vi "Read Auto update indicator.vi"(8 "error in (no error)":errorcluster, 11 "D_Datagrid in":refnum<class "D_Datagrid.lvclass">) -> (0 "error out":errorcluster, 2 "Auto-update indicator":bool, 3 "D_Datagrid out":refnum<class "D_Datagrid.lvclass">)   [LabVIEW 2018, in "D Datagrid Library.lvlib" / "D_Datagrid.lvclass"]
uses:
  D_Datagrid.lvclass
  D_Datagrid.lvclass/D_Datagrid.ctl
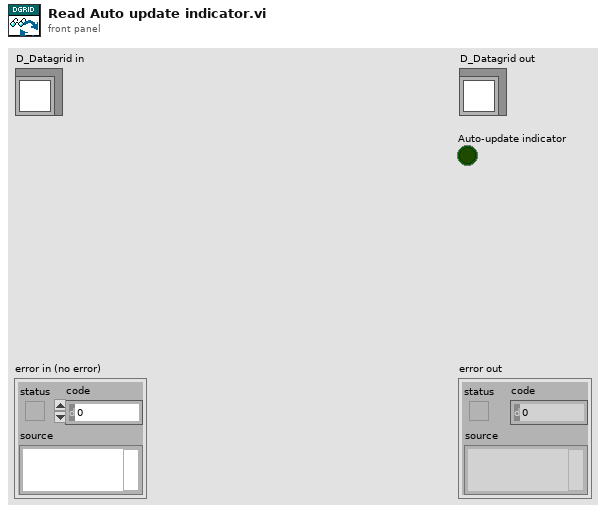
[diagram p1: front panel]
types:
  T1 = typedef "D Datagrid Library.lvlib/D_Datagrid.lvclass/State Data.ctl" = cluster{"Data elements":refnum<class "DatagridElement.lvclass">[][], "Auto-update indicator":bool}
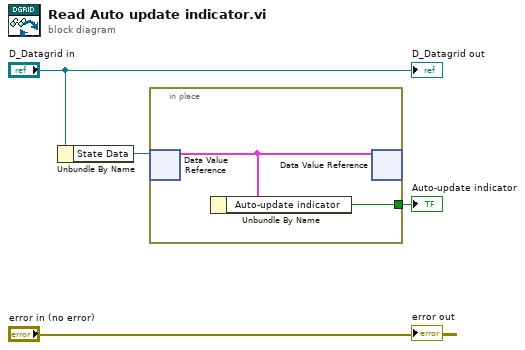
[diagram p0: block diagram]
diagram:
  n1 = Unbundle By Name("D_Datagrid in") -> ("State Data"=w4:refnum<data-value>)
  n2 = in-place {
    in-place-border: [w5] -> w3
    n3 = in-place-dvr #1(w4) -> (w6:T1)  [unwired: 1 out]
    n4 = Unbundle By Name(w6) -> ("Auto-update indicator"=w5:bool)
    n5 = in-place-dvr #1(w6) -> ()  [unwired: 2 out]
  }
  "Auto-update indicator" <- w3
  "error out" <- "error in (no error)"
  "D_Datagrid out" <- "D_Datagrid in"
